vi "QI_ConfigCam.vi"(0 "Camera Handle":u32, 2 "Parameter":T2, 3 "paramVal":u32, 4 "Readout Speed":T1, 5 "error in (no error)":errorcluster, 7 "High Sensitivity":bool=TRUE, 8 "path to dll":path, 9 "CCD Width":u32, 11 "CCD Height":u32) -> (14 "Camera Handle":u32, 17 "ConfigCam err":i32, 19 "error out":errorcluster)   [LabVIEW 2014]
uses:
  Controls/Parameter.ctl
  Controls/Readout Speed.ctl
  Release/QImaging.dll
panel:
  in  "paramKey":u32
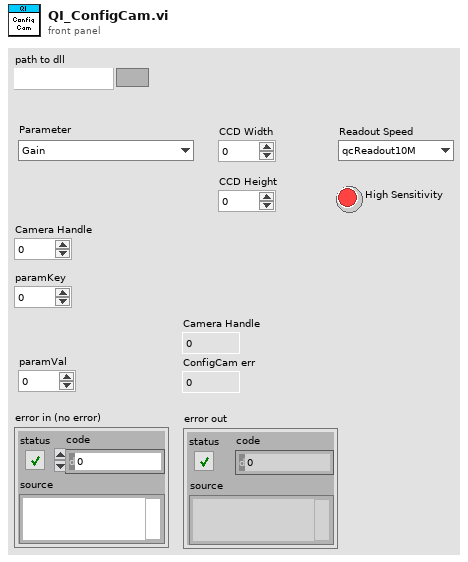
[diagram p1: front panel]
types:
  T1 = typedef "Readout Speed.ctl" = enum16{"qcReadout10M", "qcReadout20M", "qcReadout30M"}
  T2 = typedef "Parameter.ctl" = enum32{"Gain ", "Offset", "Exposure", "Binning", "HzBinning", "VtBinning", "Readout speed", "Trigger Type", "Color Wheel", "Cooler Active", "Exposure red", "Exposure blue", "Image format", "ROI X", "ROI Y", "ROI Width", "ROI Height", "Reserved1", "Shutter State", "Reserved2", "SyncB", "Reserved3", "IntensifierGain (deprecated)", "Trig Delay", "Camera Mode", "Normalized Gain", "Normalized Intensifier Gain", "Do post processing ", "Post Proc Gain Red", "Post Proc Gain Green", "Post Proc Gain Blue", "Post Proc Bayer Algo", "Post Proc Image Format", "Fan Speed", "Blackout Mode", "High Sensitivity Mode", "Readout Port", "EM Gain", "Open Delay Shutter", "Close Delay Shutter", "CCD Clearing Mode", "Over Sample", "Reserved5", "Reserved6", "Reserved7"}
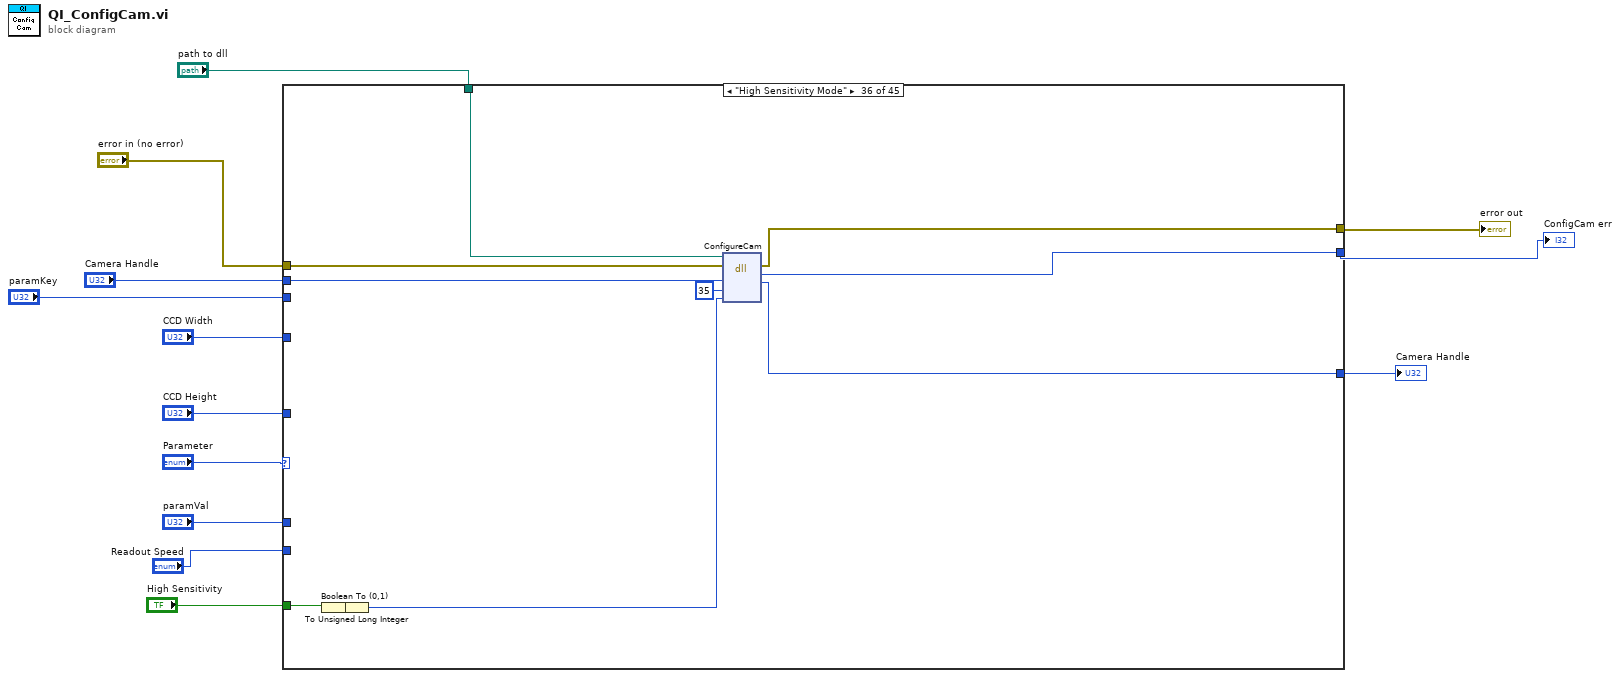
[diagram p0: block diagram]
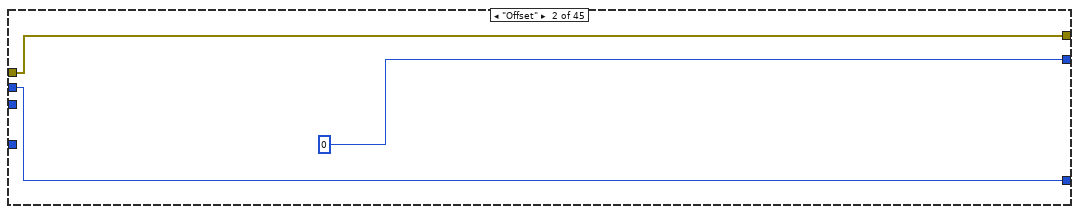
[diagram p3: hidden frame]
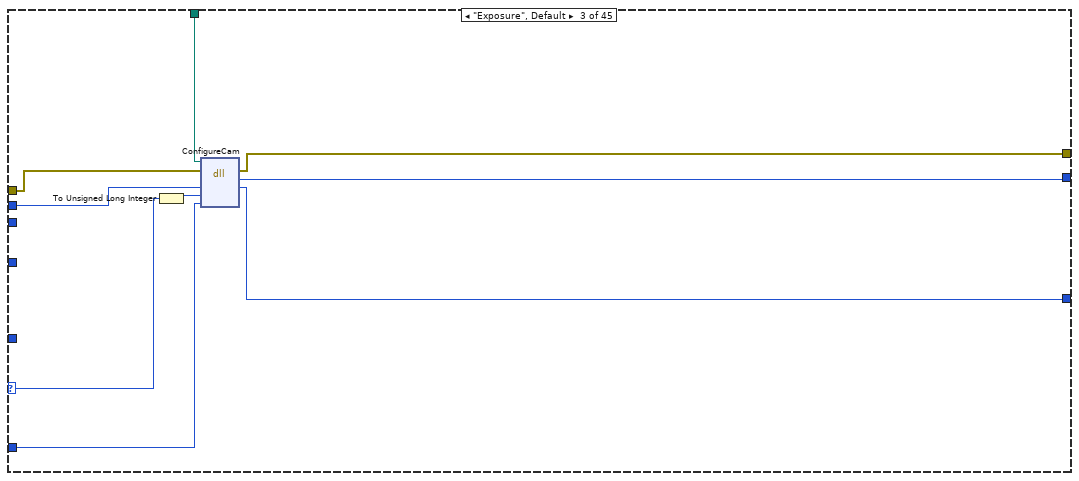
[diagram p4: hidden frame]
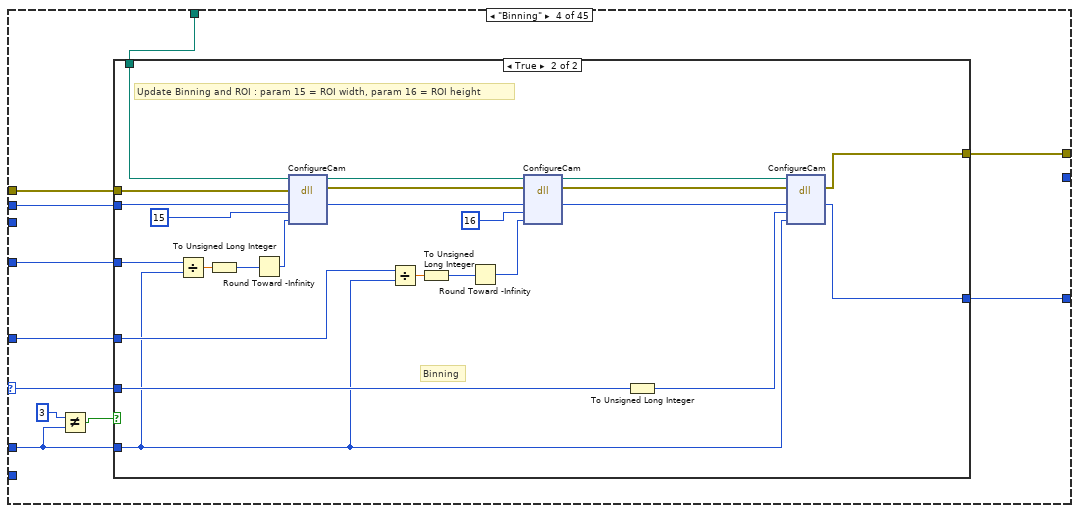
[diagram p5: hidden frame]
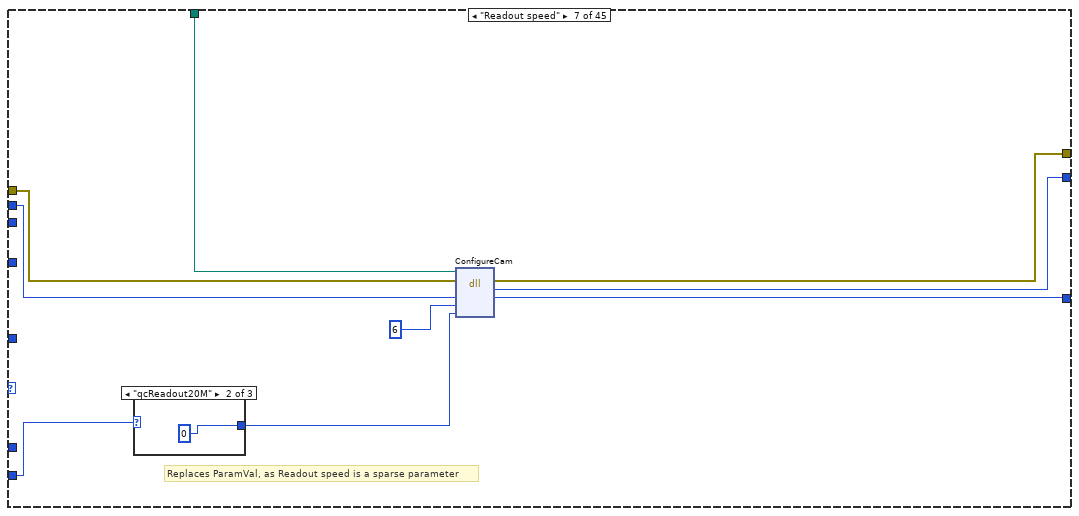
[diagram p9: hidden frame]
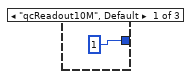
[diagram p10: hidden frame]
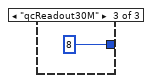
[diagram p11: hidden frame]
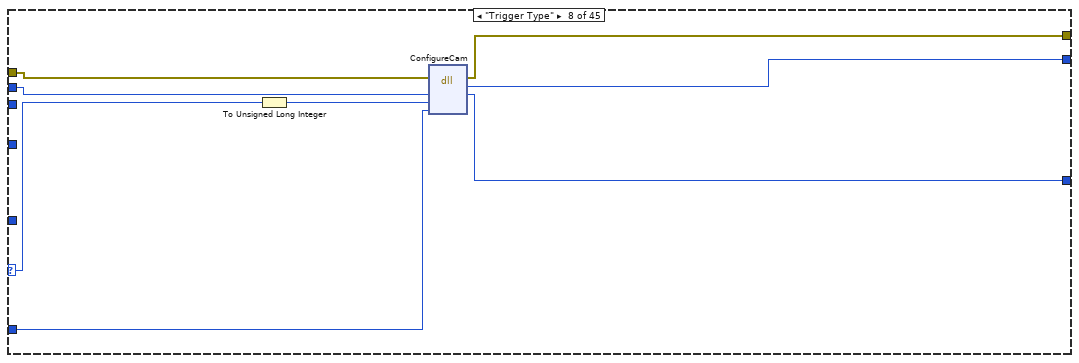
[diagram p12: hidden frame]
diagram:
  n1 = case shown="\"High Sensitivity Mode\"" "Parameter" {
    selector: "Parameter" -> [_ _ w22 w32 _ _ _ w83 _ _ _ _ _ _ _ _ _ _ _ _ _ _ _ _ _ _ _ _ _ _ _ _ _ _ _ _ _ _ _ _ _ _ _ _ _]
    tunnel: "error in (no error)" -> [w15 w18 w27 w37 w66 w68 w74 w88 w90 w92 w94 w96 w98 w100 w102 w104 w106 w108 w110 w112 w114 w116 w118 w120 w122 w124 w126 w128 w130 w132 w134 w136 w138 w140 w142 w151 w154 w156 w158 w160 w162 w164 w166 w168 w170]
    tunnel: [w15 w18 w25 w36 w66 w68 w69 w87 w90 w92 w94 w96 w98 w100 w102 w104 w106 w108 w110 w112 w114 w116 w118 w120 w122 w124 w126 w128 w130 w132 w134 w136 w138 w140 w142 w145 w154 w156 w158 w160 w162 w164 w166 w168 w170] -> w12
    tunnel: "Camera Handle" -> [w14 w17 w26 w38 w65 w67 w76 w86 w89 w91 w93 w95 w97 w99 w101 w103 w105 w107 w109 w111 w113 w115 w117 w119 w121 w123 w125 w127 w129 w131 w133 w135 w137 w139 w141 w150 w153 w155 w157 w159 w161 w163 w165 w167 w169]
    tunnel: "paramVal" -> [_ _ w24 w35 _ _ _ w82 _ _ _ _ _ _ _ _ _ _ _ _ _ _ _ _ _ _ _ _ _ _ _ _ _ _ _ _ _ _ _ _ _ _ _ _ _]
    tunnel: "paramKey" -> [_ _ _ _ _ _ _ _ _ _ _ _ _ _ _ _ _ _ _ _ _ _ _ _ _ _ _ _ _ _ _ _ _ _ _ _ _ _ _ _ _ _ _ _ _]
    tunnel: [w14 w17 w21 w29 w65 w67 w71 w85 w89 w91 w93 w95 w97 w99 w101 w103 w105 w107 w109 w111 w113 w115 w117 w119 w121 w123 w125 w127 w129 w131 w133 w135 w137 w139 w141 w143 w153 w155 w157 w159 w161 w163 w165 w167 w169] -> w7
    tunnel: [_ 0 w20 _ _ _ w70 w84 _ _ _ _ _ _ _ _ _ _ _ _ _ _ _ _ _ _ _ _ _ _ _ _ _ _ _ w144 _ _ _ _ _ _ _ _ _] -> w6
    tunnel: "CCD Width" -> [_ _ _ w31 _ _ _ _ _ _ _ _ _ _ _ _ _ _ _ _ _ _ _ _ _ _ _ _ _ _ _ _ _ _ _ _ _ _ _ _ _ _ _ _ _]
    tunnel: "CCD Height" -> [_ _ _ w30 _ _ _ _ _ _ _ _ _ _ _ _ _ _ _ _ _ _ _ _ _ _ _ _ _ _ _ _ _ _ _ _ _ _ _ _ _ _ _ _ _]
    tunnel: "path to dll" -> [_ _ w19 w28 _ _ w75 _ _ _ _ _ _ _ _ _ _ _ _ _ _ _ _ _ _ _ _ _ _ _ _ _ _ _ _ w152 _ _ _ _ _ _ _ _ _]
    tunnel: "Readout Speed" -> [_ _ _ _ _ _ w77 _ _ _ _ _ _ _ _ _ _ _ _ _ _ _ _ _ _ _ _ _ _ _ _ _ _ _ _ _ _ _ _ _ _ _ _ _ _]
    tunnel: "High Sensitivity" -> [_ _ _ _ _ _ _ _ _ _ _ _ _ _ _ _ _ _ _ _ _ _ _ _ _ _ _ _ _ _ _ _ _ _ _ w148 _ _ _ _ _ _ _ _ _]
    frame "Gain " {
    }
    frame "Offset" {
    }
    frame "Exposure", Default {
      n2 = To Unsigned Long Integer(number=w22) -> (unsigned 32bit integer=w23:u32)
      n3 = dll-call lib="C:/Users/appli/Documents/Aline/octo-labview/QImaging/Release/QImaging.dll" fn="ConfigureCam"(path in=w19, error in=w27, "handle"=w26, "paramKey"=w23, "paramVal"=w24) -> (error out=w25:errorcluster, "return type"=w20:i32, "handle"=w21:u32)  [unwired: 3 in, 1 out]
    }
    frame "Binning" {
      n4 = Not Equal?(x=u32 3, y=w35) -> (x != y?=w33:bool)
      n5 = case shown="True" w33 {
        tunnel: w38 -> [w39 w64]
        tunnel: w37 -> [w40 w63]
        tunnel: w35 -> [_ w48]
        tunnel: [w40 w60] -> w36
        tunnel: w32 -> [_ w51]
        tunnel: w31 -> [_ w55]
        tunnel: w30 -> [_ w52]
        tunnel: [w39 w49] -> w29
        tunnel: w28 -> [_ w43]
        frame False {
        }
        frame True {
          # "Binning"
          # "Update Binning and ROI : param 15 = ROI width, param 16 = ROI height"
          n6 = Divide(x=w55, y=w48) -> (x/y=w54:dbl)
          n7 = To Unsigned Long Integer(number=w54) -> (unsigned 32bit integer=w45:u32)
          n8 = Round Toward -Infinity(1:w45) -> (0:w44:u32)
          n9 = dll-call lib="C:/Users/appli/Documents/Aline/octo-labview/QImaging/Release/QImaging.dll" fn="ConfigureCam"(path in=w43, error in=w63, "handle"=w64, "paramKey"=u32 15, "paramVal"=w44) -> (path out=w42:path, error out=w62:errorcluster, "handle"=w57:u32)  [unwired: 4 in]
          n10 = Divide(x=w52, y=w48) -> (x/y=w53:dbl)
          n11 = To Unsigned Long Integer(number=w53) -> (unsigned 32bit integer=w47:u32)
          n12 = Round Toward -Infinity(1:w47) -> (0:w46:u32)
          n13 = dll-call lib="C:/Users/appli/Documents/Aline/octo-labview/QImaging/Release/QImaging.dll" fn="ConfigureCam"(path in=w42, error in=w62, "handle"=w57, "paramKey"=u32 16, "paramVal"=w46) -> (path out=w41:path, error out=w61:errorcluster, "handle"=w58:u32)  [unwired: 4 in]
          n14 = To Unsigned Long Integer(number=w51) -> (unsigned 32bit integer=w59:u32)
          n15 = dll-call lib="C:/Users/appli/Documents/Aline/octo-labview/QImaging/Release/QImaging.dll" fn="ConfigureCam"(path in=w41, error in=w61, "handle"=w58, "paramKey"=w59, "paramVal"=w48) -> (error out=w60:errorcluster, "handle"=w49:u32)  [unwired: 4 in, 1 out]
        }
      }
    }
    frame "HzBinning" {
    }
    frame "VtBinning" {
    }
    frame "Readout speed" {
      # "Replaces ParamVal, as Readout speed is a sparse parameter"
      n16 = case shown="\"qcReadout20M\"" w77 {
        tunnel: [u32 1 u32 0 u32 8] -> w73
        frame "qcReadout10M", Default {
        }
        frame "qcReadout20M" {
        }
        frame "qcReadout30M" {
        }
      }
      n17 = dll-call lib="C:/Users/appli/Documents/Aline/octo-labview/QImaging/Release/QImaging.dll" fn="ConfigureCam"(path in=w75, error in=w74, "handle"=w76, "paramKey"=u32 6, "paramVal"=w73) -> (error out=w69:errorcluster, "return type"=w70:i32, "handle"=w71:u32)  [unwired: 3 in, 1 out]
    }
    frame "Trigger Type" {
      n18 = To Unsigned Long Integer(number=w83) -> (unsigned 32bit integer=w81:u32)
      n19 = dll-call lib="Z:/Programmes en Developpement/QImaging/Release/QImaging.dll" fn="ConfigureCam"(error in=w88, "handle"=w86, "paramKey"=w81, "paramVal"=w82) -> (error out=w87:errorcluster, "return type"=w84:i32, "handle"=w85:u32)  [unwired: 4 in, 1 out]
    }
    frame "Color Wheel" {
    }
    frame "Cooler Active" {
    }
    frame "Exposure red" {
    }
    frame "Exposure blue" {
    }
    frame "Image format" {
    }
    frame "ROI X" {
    }
    frame "ROI Y" {
    }
    frame "ROI Width" {
    }
    frame "ROI Height" {
    }
    frame "Reserved1" {
    }
    frame "Shutter State" {
    }
    frame "Reserved2" {
    }
    frame "SyncB" {
    }
    frame "Reserved3" {
    }
    frame "IntensifierGain (deprecated)" {
    }
    frame "Trig Delay" {
    }
    frame "Camera Mode" {
    }
    frame "Normalized Gain" {
    }
    frame "Normalized Intensifier Gain" {
    }
    frame "Do post processing " {
    }
    frame "Post Proc Gain Red" {
    }
    frame "Post Proc Gain Green" {
    }
    frame "Post Proc Gain Blue" {
    }
    frame "Post Proc Bayer Algo" {
    }
    frame "Post Proc Image Format" {
    }
    frame "Fan Speed" {
    }
    frame "Blackout Mode" {
    }
    frame "High Sensitivity Mode" {
      n20 = Boolean To (0,1)(Boolean=w148) -> (0, 1=w147:i16)
      n21 = To Unsigned Long Integer(number=w147) -> (unsigned 32bit integer=w146:u32)
      n22 = dll-call lib="C:/Users/appli/Documents/Aline/octo-labview/QImaging/Release/QImaging.dll" fn="ConfigureCam"(path in=w152, error in=w151, "handle"=w150, "paramKey"=u32 35, "paramVal"=w146) -> (error out=w145:errorcluster, "return type"=w144:i32, "handle"=w143:u32)  [unwired: 3 in, 1 out]
    }
    frame "Readout Port" {
    }
    frame "EM Gain" {
    }
    frame "Open Delay Shutter" {
    }
    frame "Close Delay Shutter" {
    }
    frame "CCD Clearing Mode" {
    }
    frame "Over Sample" {
    }
    frame "Reserved5" {
    }
    frame "Reserved6" {
    }
    frame "Reserved7" {
    }
  }
  "error out" <- w12
  "Camera Handle" <- w7
  "ConfigCam err" <- w6
